vi "Write equipoSeleccionado.vi"(8 "error in (no error)":errorcluster, 10 "equipoSeleccionado":string, 11 "Equipo in":refnum<class "Equipo.lvclass">) -> (0 "error out":errorcluster, 3 "Equipo out":refnum<class "Equipo.lvclass">)   [LabVIEW 2019, in "Equipo.lvclass"]
uses:
  Equipo.lvclass
  Equipo.lvclass/Equipo.ctl
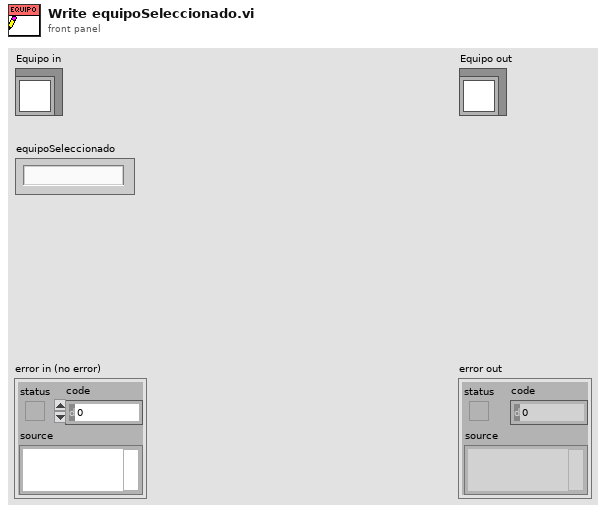
[diagram p1: front panel]
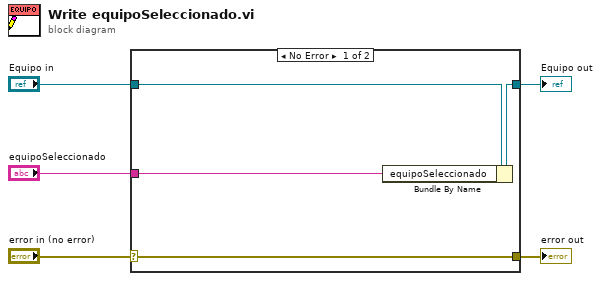
[diagram p0: block diagram]
diagram:
  n1 = case shown="No Error" "error in (no error)" {
    selector: "error in (no error)" -> [w9 w10]
    tunnel: [w9 w10] -> w4
    tunnel: [w7 w11] -> w2
    tunnel: "Equipo in" -> [w8 w11]
    tunnel: "equipoSeleccionado" -> [w6 _]
    frame No Error {
      n2 = Bundle By Name(cluster=w8, "equipoSeleccionado"=w6) -> (w7:refnum<class "Equipo.lvclass">)
    }
    frame Error {
    }
  }
  "error out" <- w4
  "Equipo out" <- w2
